vi "Set Ctl Value.vi"(8 "error in (no error)":errorcluster, 9 "Signaling?":bool, 10 "String":string, 11 "Ring Field in":refnum<class "Ring Field.lvclass">) -> (0 "error out":errorcluster, 3 "Ring Field out":refnum<class "Ring Field.lvclass">)   [LabVIEW 2020, in "Ring Field.lvclass"]
uses:
  Ring Field.lvclass
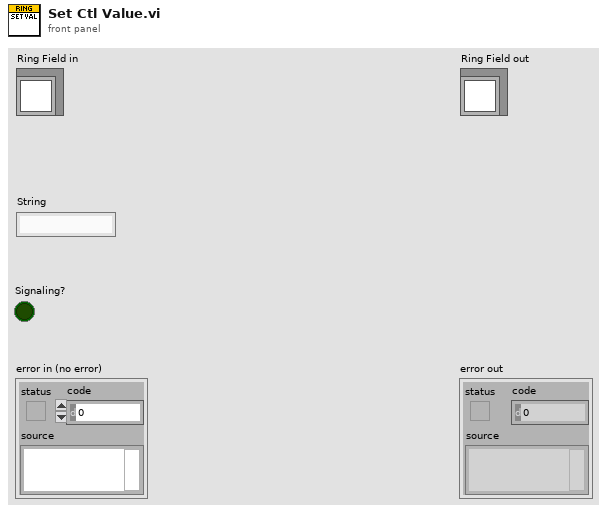
[diagram p1: front panel]
types:
  T1 = typedef "LVStringsAndValuesArrayTypeDef.ctl" = cluster{"String":string, "Value":ext}[]
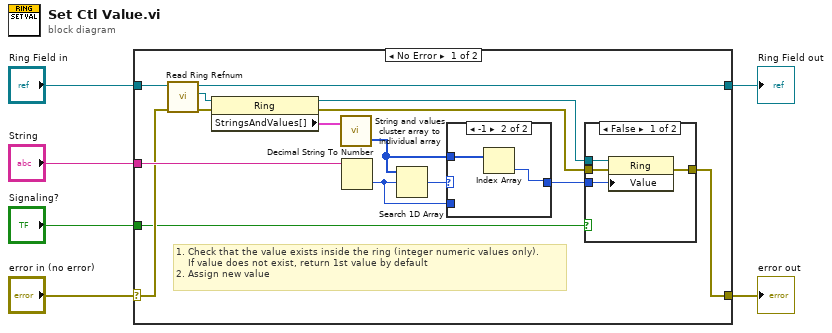
[diagram p0: block diagram]
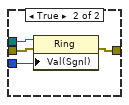
[diagram p2: hidden frame]
diagram:
  n1 = case shown="No Error" "error in (no error)" {
    selector: "error in (no error)" -> [w14 w33]
    tunnel: "Ring Field in" -> [w21 w34]
    tunnel: [w20 w34] -> w4
    tunnel: [w7 w33] -> w3
    tunnel: "String" -> [w17 _]
    tunnel: "Signaling?" -> [w11 _]
    frame No Error {
      # "1. Check that the value exists inside the ring (integer numeric values only).\n    If value does not exist, return 1st value by default\n2. Assign new value"
      n2 = call "Read Ring Refnum.vi"("error in (no error)"=w14, "Ring Field in"=w21) -> ("error out"=w16:errorcluster, "Ring Refnum"=w19:refnum<vi>, "Ring Field out"=w20:refnum<class "Ring Field.lvclass">)  [unwired: 7 in]
      n3 = property class="Ring"(reference=w19, error in=w16) -> (reference out=w8:refnum<vi>, error out=w9:errorcluster, "StringsAndValues[]"=w18:T1)
      n4 = call "String and values cluster array to individual array.vi"("Strings and Values In"=w18) -> ("Value Array Out"=w12:i32[])  [unwired: 1 out]
      n5 = Decimal String To Number(string=w17) -> (number=w13:i32)  [unwired: 2 in, 1 out]
      n6 = Search 1D Array(1D array=w12, element=w13) -> (index of element=w15:i32)  [unwired: 1 in]
      n7 = case shown="-1" w15 {
        tunnel: w13 -> [w30 _]
        tunnel: w12 -> [_ w32]
        tunnel: [w30 w31] -> w10
        frame 0, Default {
        }
        frame -1 {
          n8 = Index Array(array=w32) -> (element=w31:i32)  [unwired: 1 in]
        }
      }
      n9 = case shown="False" w11 {
        tunnel: [w25 w29] -> w7
        tunnel: w10 -> [w24 w28]
        tunnel: w9 -> [w22 w27]
        tunnel: w8 -> [w23 w26]
        frame False {
          n10 = property class="Ring"(reference=w23, error in=w22, "Value"=w24) -> (error out=w25:errorcluster)  [unwired: 1 out]
        }
        frame True {
          n11 = property class="Ring"(reference=w26, error in=w27, "Val(Sgnl)"=w28) -> (error out=w29:errorcluster)  [unwired: 1 out]
        }
      }
    }
    frame Error {
    }
  }
  "error out" <- w3
  "Ring Field out" <- w4
